vi "PDCFullInit.vi"(8 "error in (no error)":errorcluster, 11 "PDCSettings":T1) -> (0 "error out":errorcluster, 3 "DeviceNo":u32)   [LabVIEW 2015]
uses:
  TypeDefs/PDCSettings.ctl
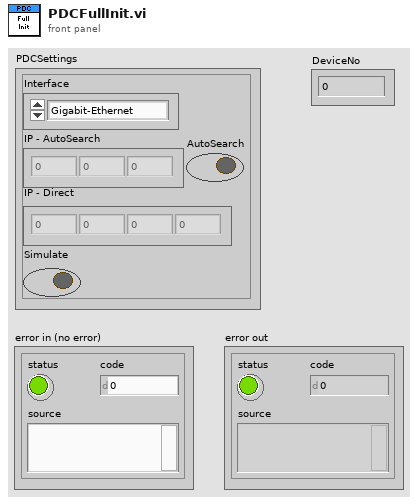
[diagram p1: front panel]
types:
  T1 = typedef "PDCSettings.ctl" = cluster{"Interface":enum16{"Gigabit-Ethernet", "IEEE1394a", "Photron Optical", "PCI/PCI Express"}, "AutoSearch":bool, "IP - AutoSearch":u32[], "IP - Direct":u32[], "Simulate":bool}
  T2 = enum16{"Gigabit-Ethernet", "IEEE1394a", "Photron Optical", "PCI/PCI Express"}
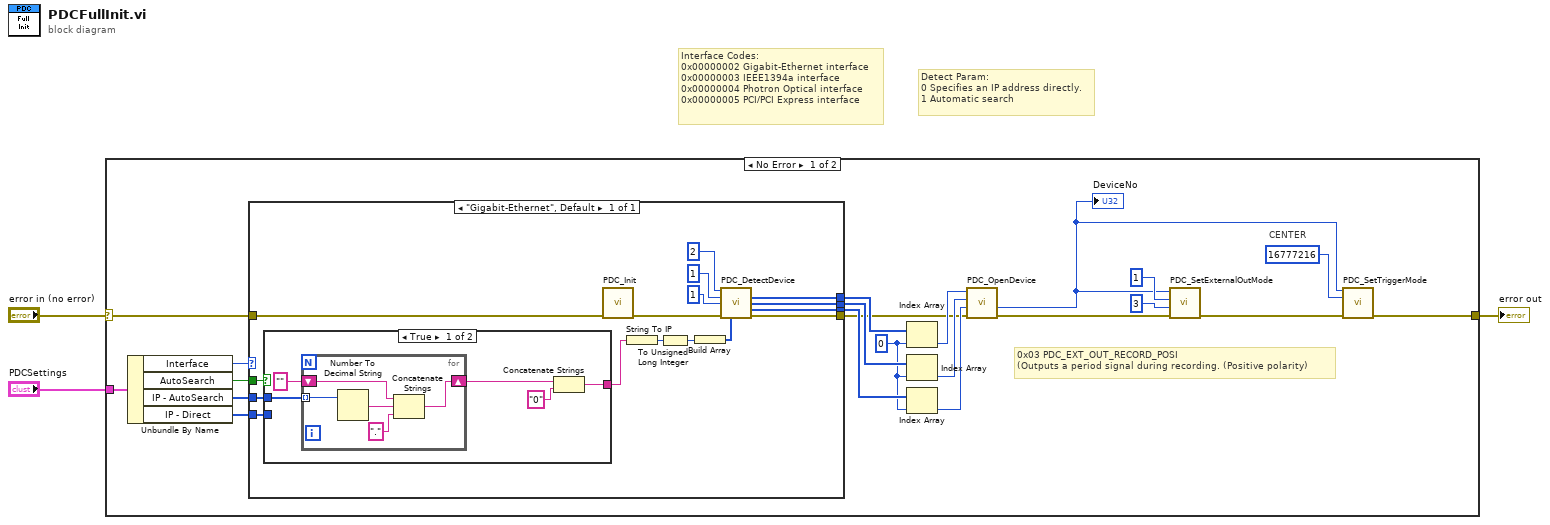
[diagram p0: block diagram]
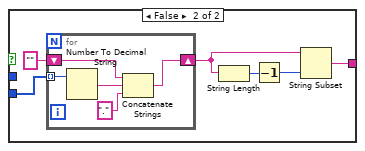
[diagram p2: hidden frame]
diagram:
  # "Detect Param:\n0 Specifies an IP address directly.\n1 Automatic search"
  # "Interface Codes:\n0x00000002 Gigabit-Ethernet interface \n0x00000003 IEEE1394a interface \n0x00000004 Photron Optical interface\n0x00000005 PCI/PCI Express interface"
  n1 = case shown="No Error" "error in (no error)" {
    selector: "error in (no error)" -> [w16 w62]
    tunnel: [w6 w62] -> w3
    tunnel: "PDCSettings" -> [w15 _]
    frame No Error {
      w18 = 0 ("Žw•W")
      # "CENTER"
      # "0x03 PDC_EXT_OUT_RECORD_POSI \n(Outputs a period signal during recording. (Positive polarity)"
      n2 = Unbundle By Name(w15) -> ("Interface"=w14:T2, "AutoSearch"=w13:bool, "IP - AutoSearch"=w12:u32[], "IP - Direct"=w11:u32[])
      n3 = case shown="\"Gigabit-Ethernet\", Default" w14 {
        tunnel: [w40] -> w21
        tunnel: [w39] -> w20
        tunnel: [w38] -> w19
        tunnel: [w37] -> w17
        tunnel: w16 -> [w29]
        tunnel: w13 -> [w28]
        tunnel: w12 -> [w27]
        tunnel: w11 -> [w25]
        frame "Gigabit-Ethernet", Default {
          n4 = case shown="True" w28 {
            tunnel: w27 -> [w45 _]
            tunnel: [w41 w54] -> w26
            tunnel: w25 -> [_ w55]
            frame True {
              n5 = for {
                tunnel: w45 -> [w50] mode=indexing
                shift-right: [w47] -> w43
                shift-left: "" -> [w46]
                n6 = Number To Decimal String(number=w50) -> (decimal integer string=w49:string)  [unwired: 1 in]
                n7 = Concatenate Strings(w46, w49, "." ("element")) -> (w47:string)
              }
              n8 = Concatenate Strings(w43, "0" ("string")) -> (w41:string)
            }
            frame False {
              n9 = for {
                tunnel: w55 -> [w61] mode=indexing
                shift-right: [w58] -> w53
                shift-left: "" -> [w57]
                n10 = Number To Decimal String(number=w61) -> (decimal integer string=w60:string)  [unwired: 1 in]
                n11 = Concatenate Strings(w57, w60, "." ("element")) -> (w58:string)
              }
              n12 = String Length(string=w53) -> (length=w52:i32)
              n13 = Decrement(x=w52) -> (x-1=w51:i32)
              n14 = String Subset(string=w53, length (rest)=w51) -> (substring=w54:string)  [unwired: 1 in]
            }
          }
          n15 = call "PDC_Init.vi"("error in (no error)"=w29) -> ("error out"=w30:errorcluster)  [unwired: 8 in, 2 out]
          n16 = String To IP(1:w26) -> (0:w34:u32)
          n17 = To Unsigned Long Integer(number=w34) -> (unsigned 32bit integer=w35:u32)
          n18 = Build Array(w35) -> (w36:u32[])
          n19 = call "PDC_DetectDevice.vi"("InterfaceCode"=u32 2, "DetectNum"=u32 1, "DetectParam"=u32 1, "error in (no error)"=w30, "DetectNo"=w36) -> ("DeviceCode"=w38:u32[], "TmpDeviceNo"=w39:u32[], "InterfaceCode(out)"=w40:u32[], "error out"=w37:errorcluster)  [unwired: 4 in, 3 out]
        }
      }
      n20 = Index Array(array=w19, index=w18) -> (element=w22:u32)
      n21 = Index Array(array=w20, index=w18) -> (element=w23:u32)
      n22 = Index Array(array=w21, index=w18) -> (element=w24:u32)
      n23 = call "PDC_OpenDevice.vi"("error in (no error)"=w17, "InterfaceCode"=w24, "TmpDeviceNo"=w23, "DeviceCode"=w22) -> ("error out"=w10:errorcluster, "DeviceNo"=w5:u32)  [unwired: 4 in, 2 out]
      "DeviceNo" <- w5
      n24 = call "PDC_SetExternalOutMode.vi"("error in (no error)"=w10, "Mode"=u32 3, "Port"=u32 1, "DeviceNo"=w5) -> ("error out"=w7:errorcluster)  [unwired: 5 in, 2 out]
      n25 = call "PDC_SetTriggerMode.vi"("DeviceNo"=w5, "Mode"=u32 16777216 ("nMode"), "error in (no error)"=w7) -> ("error out"=w6:errorcluster)  [unwired: 10 in, 2 out]
    }
    frame Error {
    }
  }
  "error out" <- w3
